vi "SubscriberRequestTopic.vi"(3 "LogPath in":path, 4 "ROS":T1, 5 "Node URI":string) -> (0 "LogPath out":path, 1 "Topic Request Reply":T3, 2 "Topic URI":string)   [LabVIEW 2012]
doc: "Asks the node to get a publisher node from the master and replies with the port"
uses:
  <userlib>/ROS for LabVIEW Software/ROS/Code/SubVIs/_ROSControl.ctl
  <userlib>/ROS for LabVIEW Software/ROS/Code/SubVIs/_ROSDirection.ctl
  <userlib>/ROS for LabVIEW Software/ROS/Code/_ROSDefinition.vi
panel:
  out "error out":errorcluster
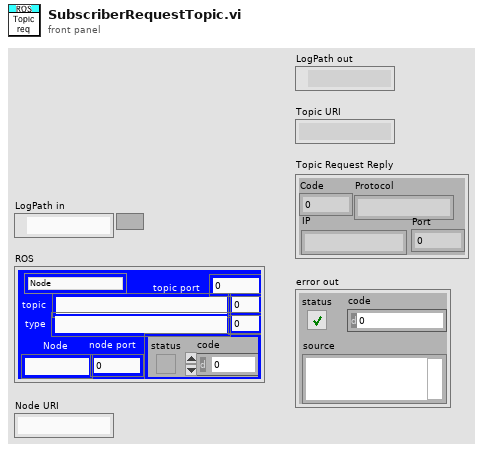
[diagram p1: front panel]
types:
  T1 = typedef "_ROSControl.ctl" = cluster{"topic port":u16, "Node":string, "topic":string, "type":string, "node port":u16, "error ":errorcluster, "Direction":T2, "Update (ms)":u16, "FIFO size":u16}
  T2 = typedef "_ROSDirection.ctl" = enum16{"Node", "Publisher", "Subscriber", "ServiceClient", "ServiceProvider"}
  T3 = cluster{"Protocol":string, "Code":i32, "IP":string, "Port":i32}
  T4 = cluster{"Code":i32, "Status Message":string, "APIs":string[]}
  T5 = typedef "ROSLog.ctl" = cluster{"Sent":string, "Reply":string, "MethodName":string, "success":bool, "Dir1":string, "Dir2":string, "Time Stamp":string, "error":errorcluster, "Preamble":string, "Midamble":string, "Postamble":string}
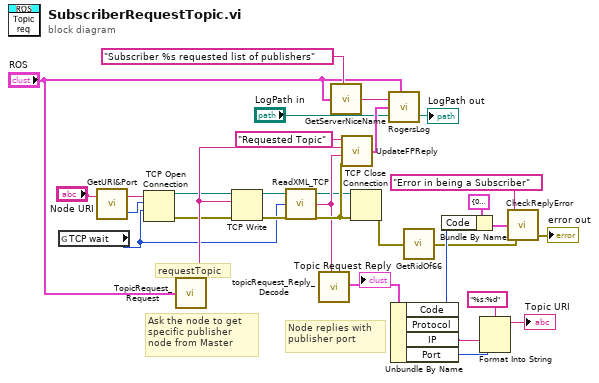
[diagram p0: block diagram]
diagram:
  # "requestTopic"
  # "Node replies with publisher port"
  # "Ask the node to get specific publisher node from Master"
  n1 = global read "_ROSDefinition.vi" "TCP wait"() -> (w1:i32)
  n2 = call <userlib>:"GetURI&Port.vi"("URI in"="Node URI") -> ("Port"=w16:u16, "URI"=w15:string)
  n3 = TCP Open Connection(address=w15, remote port or service name=w16, timeout ms (60000)=w1) -> (connection ID=w4:refnum<k5>, error out=w3:errorcluster)  [unwired: 2 in]
  n4 = call <userlib>:"TopicRequest_Request.vi"("ROS"="ROS") -> ("XML"=w22:string)
  n5 = TCP Write(connection ID=w4, data in=w22, error in (no error)=w3) -> (connection ID out=w5:refnum<k5>, error out=w6:errorcluster)  [unwired: 1 in, 1 out]
  n6 = call <userlib>:"ReadXML_TCP.vi"("error in"=w6, "timeout ms (3000)"=w1, "connection ID in"=w5) -> ("error out"=w24:errorcluster, "data out"=w23:string, "connection ID out"=w7:refnum<k5>)
  n7 = call <userlib>:"topicRequest_Reply_Decode.vi"("Topic Request Reply"=w23) -> ("Topic Request Reply"=w8:T3)
  "Topic Request Reply" <- w8
  n8 = call <userlib>:"GetServerNiceName.vi"("ROS"="ROS", "Text to add"="Subscriber %s requested list of publishers") -> ("String"=w29:string)
  n9 = call <userlib>:"UpdateFPReply.vi"("error in (no error)"=w24, "Reply"=w23, "Sent"=w22, "method"="Requested Topic") -> ("Log"=w27:T5)
  n10 = TCP Close Connection(connection ID=w7, error in (no error)=w24) -> (error out=w9:errorcluster)  [unwired: 1 in, 1 out]
  n11 = call <userlib>:"RogersLog.vi"("Text to add"=w29, "ROS"="ROS", "Log"=w27, "LogPath in"="LogPath in") -> ("LogPath out"=→"LogPath out":path)  [unwired: 1 in, 1 out]
  n12 = Unbundle By Name(w8) -> ("Code"=w12:i32, "IP"=w20:string, "Port"=w21:i32)  [unwired: 1 out]
  n13 = call <userlib>:"GetRidOf66.vi"("error in (no error)"=w9) -> ("error out"=w11:errorcluster)
  n14 = Bundle By Name(cluster=T4 {"Code"=0, "Status Message"="", "APIs"=[]} ("Response"), "Code"=w12) -> (w14:T4)
  n15 = Format Into String(format string="%s:%d", w20, w21) -> (resulting string=→"Topic URI":string)  [unwired: 2 in, 1 out]
  n16 = call <userlib>:"CheckReplyError.vi"("error in"=w11, "Response"=w14, "Error String"="Error in being a Subscriber" ("source")) -> ("error out"=→"error out":errorcluster)  [unwired: 2 out]
